vi "File Path.vi"(11 "Program mode":string="Data") -> (3 "appended path":path)   [LabVIEW 2015]
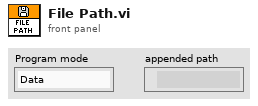
[diagram p1: front panel]
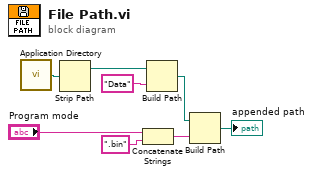
[diagram p0: block diagram]
diagram:
  n1 = call <vilib>:"Application Directory.vi"() -> ("Application Directory"=w4:path)
  n2 = Strip Path(path=w4) -> (stripped path=w5:path)  [unwired: 1 out]
  n3 = Concatenate Strings("Program mode", ".bin" ("string")) -> (w1:string)
  n4 = Build Path(base path=w5, name or relative path="Data") -> (appended path=w7:path)
  n5 = Build Path(base path=w7, name or relative path=w1) -> (appended path=→"appended path":path)
